vi "Allocate Multiple Blocks.vi"(8 "error in (no error)":errorcluster, 10 "sizes (bytes)":i32[](array[numeric]), 11 "GE 5565PIORC in":refnum<class "GE 5565PIORC.lvclass">) -> (0 "error out":errorcluster, 2 "Block Descriptors":T1[](array[typedef]) {"next descriptor ptr" format="%08x"; "data size" format="%08x"; "data ptr (upper)" format="%08x"; "data ptr (lower)" format="%08x"; "descriptor ptr (aligned)" format="%08x"; "descriptor size" format="%08x"; "descriptor ptr (VISA)" format="%08x"}, 3 "GE 5565PIORC out":refnum<class "GE 5565PIORC.lvclass">)   [LabVIEW 2016, in "GE 5565PIORC.lvclass"]
uses:
  GE 5565PIORC.lvclass
  Controls/DMA Block Descriptor.ctl
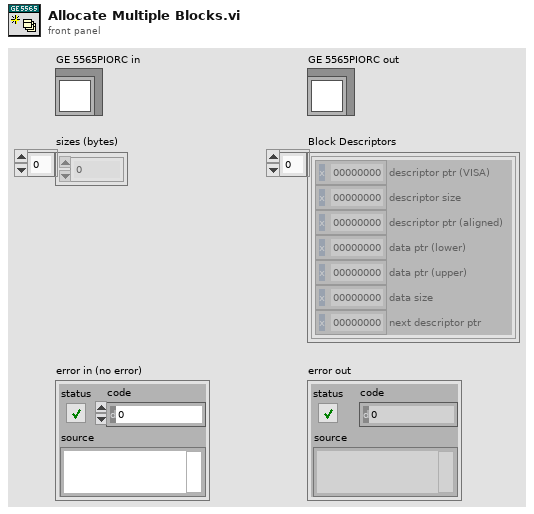
[diagram p1: front panel]
types:
  T1 = typedef "GE 5565PIORC.lvclass/DMA Block Descriptor.ctl" = cluster{"descriptor ptr (VISA)":u32, "descriptor size":u32, "descriptor ptr (aligned)":u32, "data ptr (lower)":u32, "data ptr (upper)":u32, "data size":u32, "next descriptor ptr":u32}
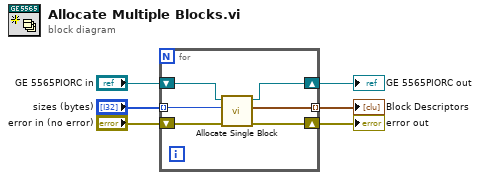
[diagram p0: block diagram]
diagram:
  n1 = for {
    tunnel: "sizes (bytes)" -> [w12] mode=indexing
    shift-right: [w10] -> w3
    shift-left: "GE 5565PIORC in" -> [w11]
    shift-right: [w8] -> w2
    shift-left: "error in (no error)" -> [w9]
    tunnel: [w7] -> w1 mode=indexing
    n2 = call "Allocate Single Block.vi"("error in (no error)"=w9, "size (bytes)"=w12, "GE 5565PIORC in"=w11) -> ("error out"=w8:errorcluster, "Block Descriptor"=w7:T1, "GE 5565PIORC out"=w10:refnum<class "GE 5565PIORC.lvclass">)  [unwired: 6 in]
  }
  "error out" <- w2
  "GE 5565PIORC out" <- w3
  "Block Descriptors" <- w1
